vi "Group ROI index by ROI type.vi"(11 "ROI data":dbl[][](array[numeric])) -> (1 "ROI indexes by type":T4, 3 "[ROI vis]":T1 {"ROI number" min=1 format="ROI %.0f"})   [LabVIEW 2017]
uses:
  Typedefs/ROI indexes by type.ctl
  Typedefs/ROI selector array-ROI vis.ctl
  xcontrol/Interface VIs/Interface typedefs/Interface-ROI selection cluster.ctl
  Typedefs/ROI ID Enum.ctl
panel:
  out "Indexes of ? (provisional)":i32[](array[numeric])
  out "Indexes of Miniscans":i32[](array[numeric])
  out "Indexes of POI":i32[](array[numeric])
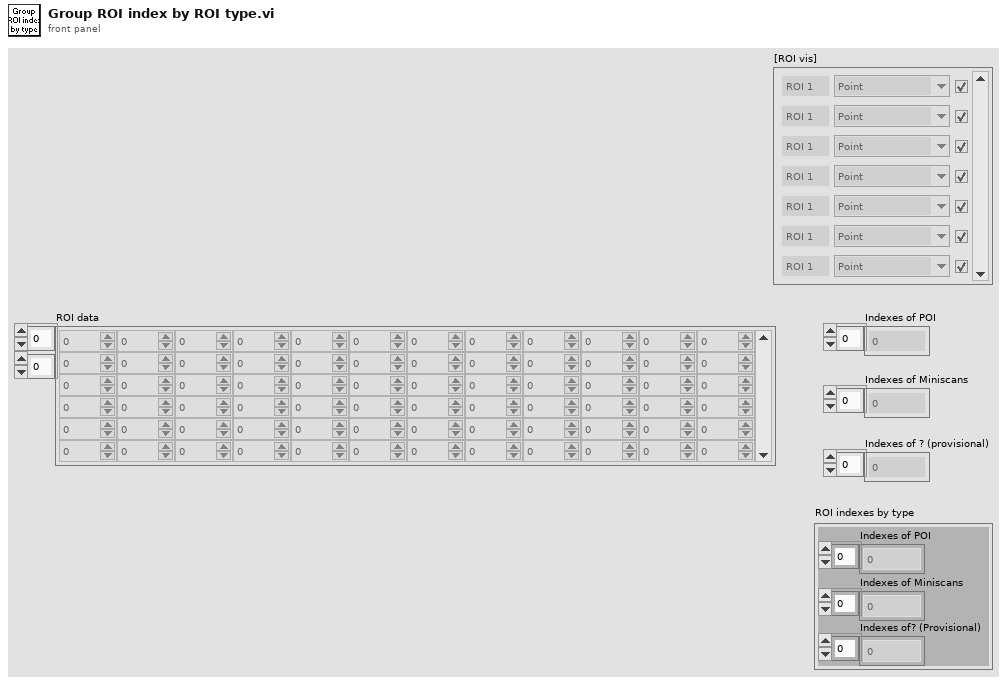
[diagram p1: front panel]
types:
  T1 = typedef "ROI selector array-ROI vis.ctl" = T2[]
  T2 = typedef "Interface-ROI selection cluster.ctl" = cluster{"ROI number":i32, "ROI ID":T3, "Visibility":bool}
  T3 = typedef "ROI ID Enum.ctl" = enum16{"Point", "MiniScan", "Comp. MiniScan", "Rectangle", "Comp. volume", "Arb. plane point"}
  T4 = typedef "ROI indexes by type.ctl" = cluster{"Indexes of POI":i32[], "Indexes of Miniscans":i32[], "Indexes of? (Provisional)":i32[]}
  T5 = typedef "ROI file columns mapping.ctl" = cluster{"\"ROI index\" column index":i32, "\"ROI ID\" column index":i32, "\"ROI Time (ns)\" column index":i32, "\"Pixels in ROI\" column index":i32, "\"X (X start)\" column index":i32, "\"Y (Y start)\" column index":i32, "\"Z (Z start)\" column index":i32, "\"X (X stop)\" column index":i32, "\"Y (Y stop)\" column index":i32, "\"Z (Z stop)\" column index":i32, "\"Angle (deg)\" column index":i32, "Composite ID":i32, "Number of lines":i32, "Frame Size":i32, "Zoom":i32, "Laser Power (%)":i32, "ROI group ID":i32}
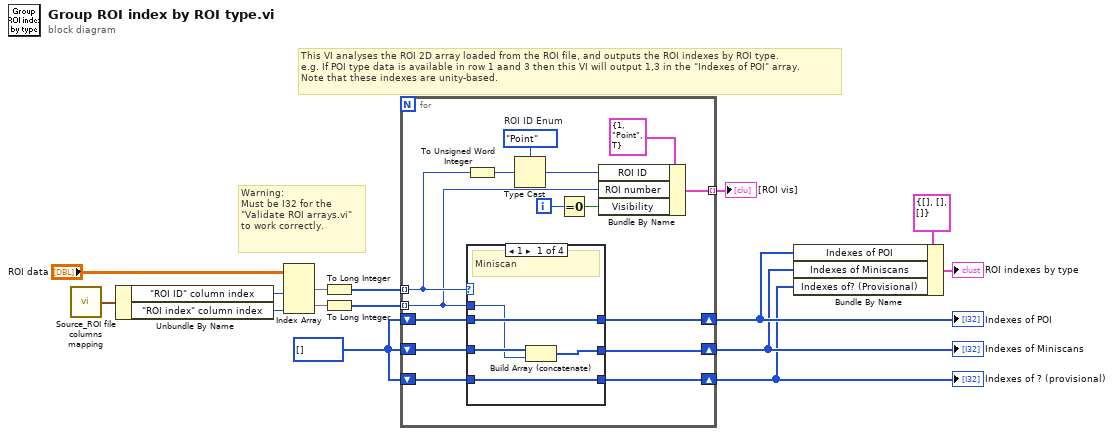
[diagram p0: block diagram]
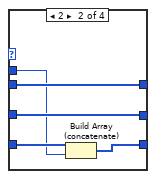
[diagram p2: hidden frame]
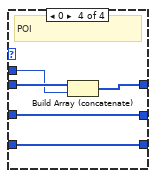
[diagram p4: hidden frame]
diagram:
  w10 = i32[] []
  # "Warning:\nMust be I32 for the \"Validate ROI arrays.vi\" to work correctly."
  # "This VI analyses the ROI 2D array loaded from the ROI file, and outputs the ROI indexes by ROI type.\ne.g. If POI type data is available in row 1 aand 3 then this VI will output 1,3 in the \"Indexes of POI\" array.\nNote that these indexes are unity-based."
  n1 = call "Source_ROI file columns mapping.vi"() -> ("ROI file columns mapping"=w9:T5)  [unwired: 1 in]
  n2 = Unbundle By Name(w9) -> ("\"ROI ID\" column index"=w8:i32, "\"ROI index\" column index"=w7:i32)
  n3 = Index Array(array="ROI data", index (col) #1=w8, index (col) #2=w7) -> (element #1=w14:dbl[], element #2=w12:dbl[])  [unwired: 2 in]
  n4 = To Long Integer(number=w14) -> (32bit integer=w13:i32[])
  n5 = To Long Integer(number=w12) -> (32bit integer=w11:i32[])
  n6 = for {
    tunnel: w11 -> [w17] mode=indexing
    shift-right: [w29] -> w4
    shift-left: w10 -> [w30]
    shift-right: [w28] -> w3
    shift-left: w10 -> [w27]
    tunnel: w13 -> [w23] mode=indexing
    shift-right: [w26] -> w2
    shift-left: w10 -> [w25]
    tunnel: [w18] -> w1 mode=indexing
    i -> [w20]
    w24 = ROI_ID_Enum."Point"  # ROI ID Enum
    n7 = To Unsigned Word Integer(number=w23) -> (unsigned 16bit integer=w16:u16)
    n8 = case shown="1" w23 {
      tunnel: w30 -> [w35 w40 w43 w48]
      tunnel: [w35 w40 w43 w47] -> w29
      tunnel: [w34 w37 w42 w46] -> w28
      tunnel: w27 -> [w33 w37 w42 w46]
      tunnel: w17 -> [w32 w36 _ w45]
      tunnel: [w31 w39 w41 w44] -> w26
      tunnel: w25 -> [w31 w38 w41 w44]
      frame 1 {
        # "Miniscan"
        n9 = Build Array (concatenate)(w33, w32) -> (w34:i32[])
      }
      frame 2 {
        n10 = Build Array (concatenate)(w38, w36) -> (w39:i32[])
      }
      frame Default {
        # "Invalid"
      }
      frame 0 {
        # "POI"
        n11 = Build Array (concatenate)(w48, w45) -> (w47:i32[])
      }
    }
    n12 = Type Cast(type=w24, x=w16) -> (*(type *) &x=w22:T3)
    n13 = Equal To 0?(x=w20) -> (x = 0?=w21:bool)
    n14 = Bundle By Name(cluster=T2 {"ROI number"=1, "ROI ID"=enum."Point", "Visibility"=TRUE} ("ROI selection cluster"), "ROI ID"=w22, "ROI number"=w17, "Visibility"=w21) -> (w18:T2)
  }
  "Indexes of POI" <- w4
  "Indexes of Miniscans" <- w3
  "Indexes of ? (provisional)" <- w2
  "[ROI vis]" <- w1
  n15 = Bundle By Name(cluster=T4 {"Indexes of POI"=[], "Indexes of Miniscans"=[], "Indexes of? (Provisional)"=[]} ("ROI indexes by type"), "Indexes of POI"=w4, "Indexes of Miniscans"=w3, "Indexes of? (Provisional)"=w2) -> (→"ROI indexes by type":T4)
